vi "Multichannel_Read.vi"(6 "WC Mode":i32=1, 8 "error in (no error)":errorcluster, 9 "Array in":u64[](array[numeric]), 10 "Cluster":T1, 11 "Refnum in":refnum<k20>) -> (0 "error out":errorcluster, 3 "Array out":u64[](array[numeric]))   [LabVIEW 2016]
uses:
  error.llb/Error Cluster From Error Code.vi
  <vilib>/rvi/errors/niLvFpgaAdjustHostInterfaceError.vi
  <vilib>/rvi/interface/nirviMethod/nirviMethod.xnode
  <vilib>/FPGAPlugInAG/Dynamic/niLvFpga_ReadFifo_Dynamic.vi
  <vilib>/rvi/errors/niLvFpgaMergeErrorWithErrorCode.vi
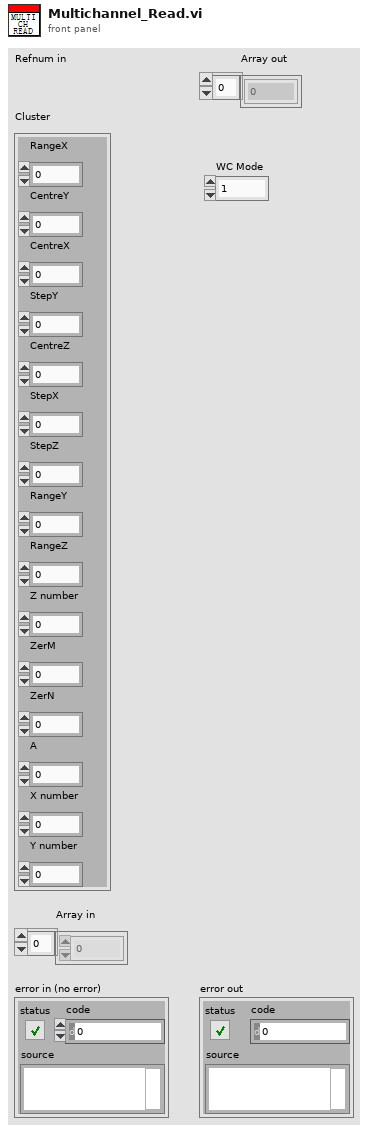
[diagram p1: front panel]
types:
  T1 = cluster{"RangeX":dbl, "CentreY":dbl, "CentreX":dbl, "StepY":dbl, "CentreZ":dbl, "StepX":dbl, "StepZ":dbl, "RangeY":dbl, "RangeZ":dbl, "Z number":i32, "ZerM":dbl, "ZerN":dbl, "A":dbl, "X number":i32, "Y number":i32}
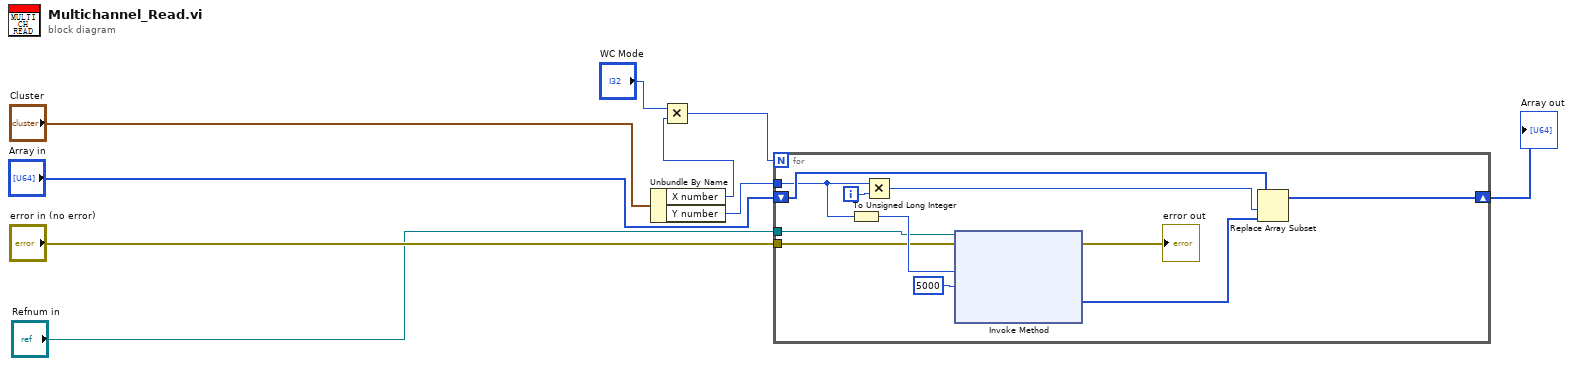
[diagram p0: block diagram]
diagram:
  n1 = Unbundle By Name("Cluster") -> ("X number"=w2:i32, "Y number"=w9:i32)
  n2 = Multiply(x="WC Mode", y=w2) -> (x*y=w1:i32)
  n3 = for {
    N: w1 -> [_]
    tunnel: "Refnum in" -> [w19]
    tunnel: "error in (no error)" -> [w18]
    shift-right: [w13] -> w7
    shift-left: "Array in" -> [w15]
    tunnel: w9 -> [w10]
    i -> [w12]
    n4 = To Unsigned Long Integer(number=w10) -> (unsigned 32bit integer=w20:u32)
    n5 = Multiply(x=w10, y=w12) -> (x*y=w11:i32)
    n6 = xnode "Invoke Method"("FPGA VI Reference In"=w19, "error in"=w18, "Number of Elements"=w20, "Timeout (ms)"=5000) -> ("error out"=→"error out":errorcluster, "Data"=w14:u64[])  [unwired: 2 out]
    n7 = Replace Array Subset(array=w15, new element=w14, index=w11) -> (w13:u64[])
  }
  "Array out" <- w7
